vi "ief_get_input_word.vi"(3 "error in (no error)":errorcluster, 4 "Input Number":u16=1 min=1 max=1024, 5 "Tagprefix in":refnum<k21>) -> (0 "error out (no error)":errorcluster, 1 "Input State":u16, 2 "Tagprefix out":refnum<k21>)   [LabVIEW 2015, in "IEF Werner.lvlib"]
doc: "The VI returns the present input word state of the chosen input word.\n\nInput Number Range:\n0001 - 0400, hex\n1 - 1024, dec"
uses:
  IEF Werner.lvlib
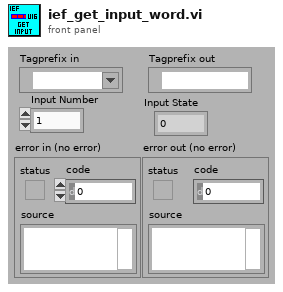
[diagram p1: front panel]
types:
  T1 = typedef "Semaphore RefNum" = refnum<k1>
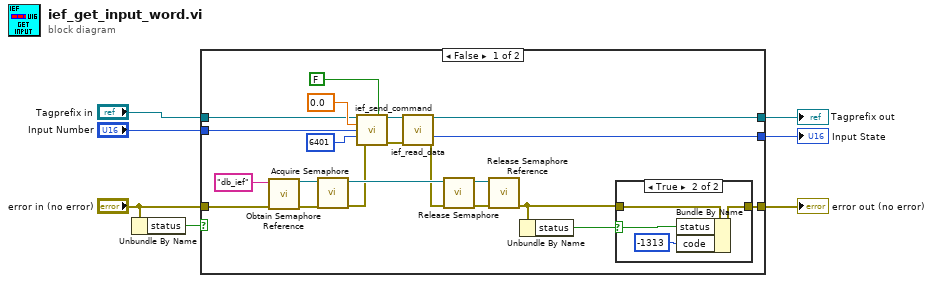
[diagram p0: block diagram]
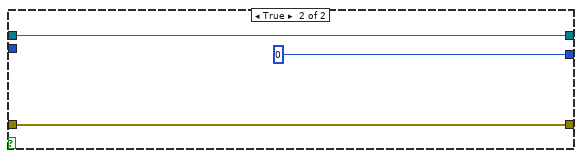
[diagram p3: hidden frame]
diagram:
  n1 = Unbundle By Name("error in (no error)") -> ("status"=w3:bool)
  n2 = case shown="False" w3 {
    tunnel: "error in (no error)" -> [w15 w36]
    tunnel: "Input Number" -> [w13 _]
    tunnel: [w25 w36] -> w6
    tunnel: [w12 u16 0 ("value uint 16")] -> w5
    tunnel: "Tagprefix in" -> [w10 w35]
    tunnel: [w8 w35] -> w1
    frame False {
      n3 = call <vilib>:"Obtain Semaphore Reference.vi"("error in (no error)"=w15, "name (unnamed)"="db_ief") -> ("error out"=w21:errorcluster, "semaphore"=w20:T1)  [unwired: 3 in, 1 out]
      n4 = call <vilib>:"Acquire Semaphore.vi"("error in (no error)"=w21, "semaphore"=w20) -> ("error out"=w18:errorcluster, "semaphore out"=w22:T1)  [unwired: 3 in, 1 out]
      n5 = call "ief_send_command.vi"("Tagprefix in"=w10, "Command datum of type real"=FALSE, "Command datum"=sgl 0.0, "Command parameter"=w13, "Command code"=u16 6401, "error in (no error)"=w18) -> ("Tagprefix out"=w9:refnum<k21>, "error out (no error)"=w26:errorcluster)  [unwired: 4 in, 4 out]
      n6 = call "ief_read_data.vi"("Tagprefix in"=w9, "error in (no error)"=w26) -> ("Tagprefix out"=w8:refnum<k21>, "value uint 16"=w12:u16, "error out (no error)"=w17:errorcluster)  [unwired: 7 in, 4 out]
      n7 = call <vilib>:"Release Semaphore.vi"("error in (no error)"=w17, "semaphore"=w22) -> ("error out"=w23:errorcluster, "semaphore out"=w24:T1)  [unwired: 4 in]
      n8 = call <vilib>:"Release Semaphore Reference.vi"("error in (no error)"=w23, "semaphore"=w24) -> ("error out"=w16:errorcluster)  [unwired: 8 in, 1 out]
      n9 = Unbundle By Name(w16) -> ("status"=w11:bool)
      n10 = case shown="True" w11 {
        selector: w11 -> [_ w30]
        tunnel: [w29 w33] -> w25
        tunnel: w16 -> [w29 w32]
        frame False {
        }
        frame True {
          n11 = Bundle By Name(cluster=w32, "status"=w30, "code"=-1313) -> (w33:errorcluster)
        }
      }
    }
    frame True {
    }
  }
  "error out (no error)" <- w6
  "Input State" <- w5
  "Tagprefix out" <- w1
